vi "Hardware Config - format and values.vi"(11 "Hardware Configuration":T4={"Dev. PC"=FALSE, "Swap XY on stage"=FALSE, "No of AOD"=0, "Computer MAC address"="", "Externalise Triggers"=FALSE, "Trigger HW config"={"Available Device List"=0, "Device Address"=""}, "DAQmx Chan"={"Pockels AO"="", "Hard shutter AO"="", "PMT AOs"="", "Galvo AOs"="", "Power meter AI"=""}, "XY stage available"=FALSE, "XY Stage"={"COM port"="", "Baudrate"=0, "Type"=""}, "Z stage available"=FALSE, "Z Stage config cluster"={"COM port"="COM7", "Baudrate"=0, "Type"=""}, "Encoder available"=FALSE, "Encoder"={"IP address"="224.0.1.103", "Port"=7000, "Wheel radius (cm)"=16.0, "Encoder Trigger"=""}, "VidRec available"=FALSE, "Cam VidRec"={"DO flag-Video record"="", "DO flag-Trial start"=""}, "Laser Power Control HW config"={"Laser Power Control"="", "Laser Power Modulation Control"=enum."NI"}, "Laser 1 available"=FALSE, "Laser 1 config cluster"={"COM port"="COM7", "Baud Rate"=0, "Type"=""}, "Prechirper 1 available"=FALSE, "Prechirper 1 config cluster"={"Type"="", "Baud Rate"=0, "COM port"="COM7"}, "Control system.FPGA available?"=FALSE, "Control Sys. HW config"={"Control system.FPGA Type"=enum."Virtex 5", "Control system.Network adapter name"="", "Control system.MAC address"="", "Control system.Ethernet Port"=0, "Control system.Ethernet Port Opened"=FALSE}, "DAQ FPGA HW Config"={"FGPA Ref"=refnum, "Target"="RIO0", "input card type"=enum."AC Card"}} {"Encoder"."Wheel radius (cm)" format="%#_13g"}) -> (0 "String":string[](array[string]), 1 "String":T1, 2 "Numeric":dbl[](array[numeric]), 3 "Numeric":T3=[{"key"="Encoder.Port", "Save?"=TRUE, "Default"=7000.0}, {"key"="Encoder.Wheel radius (cm)", "Save?"=TRUE, "Default"=16.0}, {"key"="DAQ FPGA.Input type AC/DC", "Save?"=TRUE, "Default"=1.0}, {"key"="Num AOD", "Save?"=TRUE, "Default"=4.0}, {"key"="Trigger.AvailableDeviceList", "Save?"=TRUE, "Default"=1.0}, {"key"="XY Stage.Baudrate", "Save?"=TRUE, "Default"=9600.0}, {"key"="Z Stage.Baudrate", "Save?"=TRUE, "Default"=9600.0}, {"key"="Laser.Baudrate", "Save?"=TRUE, "Default"=19200.0}, {"key"="Prechirper.Baudrate", "Save?"=TRUE, "Default"=115200.0}], 4 "Boolean":bool[](array[boolean]), 6 "Boolean":T2=[{"key"="DevPC - No hardware", "Save?"=TRUE, "Default"=FALSE}, {"key"="MC Supported", "Save?"=TRUE, "Default"=FALSE}, {"key"="Axial MC", "Save?"=TRUE, "Default"=FALSE}, {"key"="Are X Y Swapped", "Save?"=TRUE, "Default"=FALSE}, {"key"="Encoder.Available?", "Save?"=TRUE, "Default"=FALSE}, {"key"="Externalise Triggers", "Save?"=TRUE, "Default"=TRUE}, {"key"="Cam VidRec.Available", "Save?"=TRUE, "Default"=TRUE}, {"key"="Control system.Ctrl FPGA available", "Save?"=TRUE, "Default"=TRUE}, {"key"="XY Stage.Available?", "Save?"=TRUE, "Default"=TRUE}, {"key"="Z Stage.Available?", "Save?"=TRUE, "Default"=FALSE}, {"key"="Laser.Available?", "Save?"=TRUE, "Default"=TRUE}, {"key"="Prechirper.Available", "Save?"=TRUE, "Default"=TRUE}])   [LabVIEW 2017]
uses:
  Typedefs/Hardware Configuration settings.ctl
  Typedefs/Triggers HW config.ctl
  Typedefs/DAQmx physical channels cluster.ctl
  Typedefs/XY Stage config cluster.ctl
  Typedefs/Z Stage config cluster.ctl
  Typedefs/Encoder config cluster.ctl
  Typedefs/Cam VidRec HW config setup cluster.ctl
  Typedefs/Laser Power Control HW config.ctl
  Typedefs/Laser 1 config cluster.ctl
  Typedefs/PreChirper 1 config cluster.ctl
  Typedefs/Control Sys HW config cluster.ctl
  Typedefs/DAQ FPGA HW config cluster.ctl
  RIG-SPECIFIC FILES/FPGA Refs/FPGA Ref.ctl
  <vilib>/userdefined/High Color/nirio_resource_hc.ctl
  Typedefs/FPGA input type AC-DC.ctl
  Typedefs/Ini file interface (DBL).ctl
  Typedefs/Ini file interface (Boolean).ctl
  Typedefs/Ini file interface (String).ctl
panel:
  out "Boolean Default cluster":i32
  out "Boolean values":i32
  out "Numeric Values":i32
  out "Numeric Default Cluster":i32
  out "String values":i32
  out "String Default Cluster":i32
  # "Numeric Array Sizes"
  # "String Array Sizes"
  # "Boolean Array Sizes"
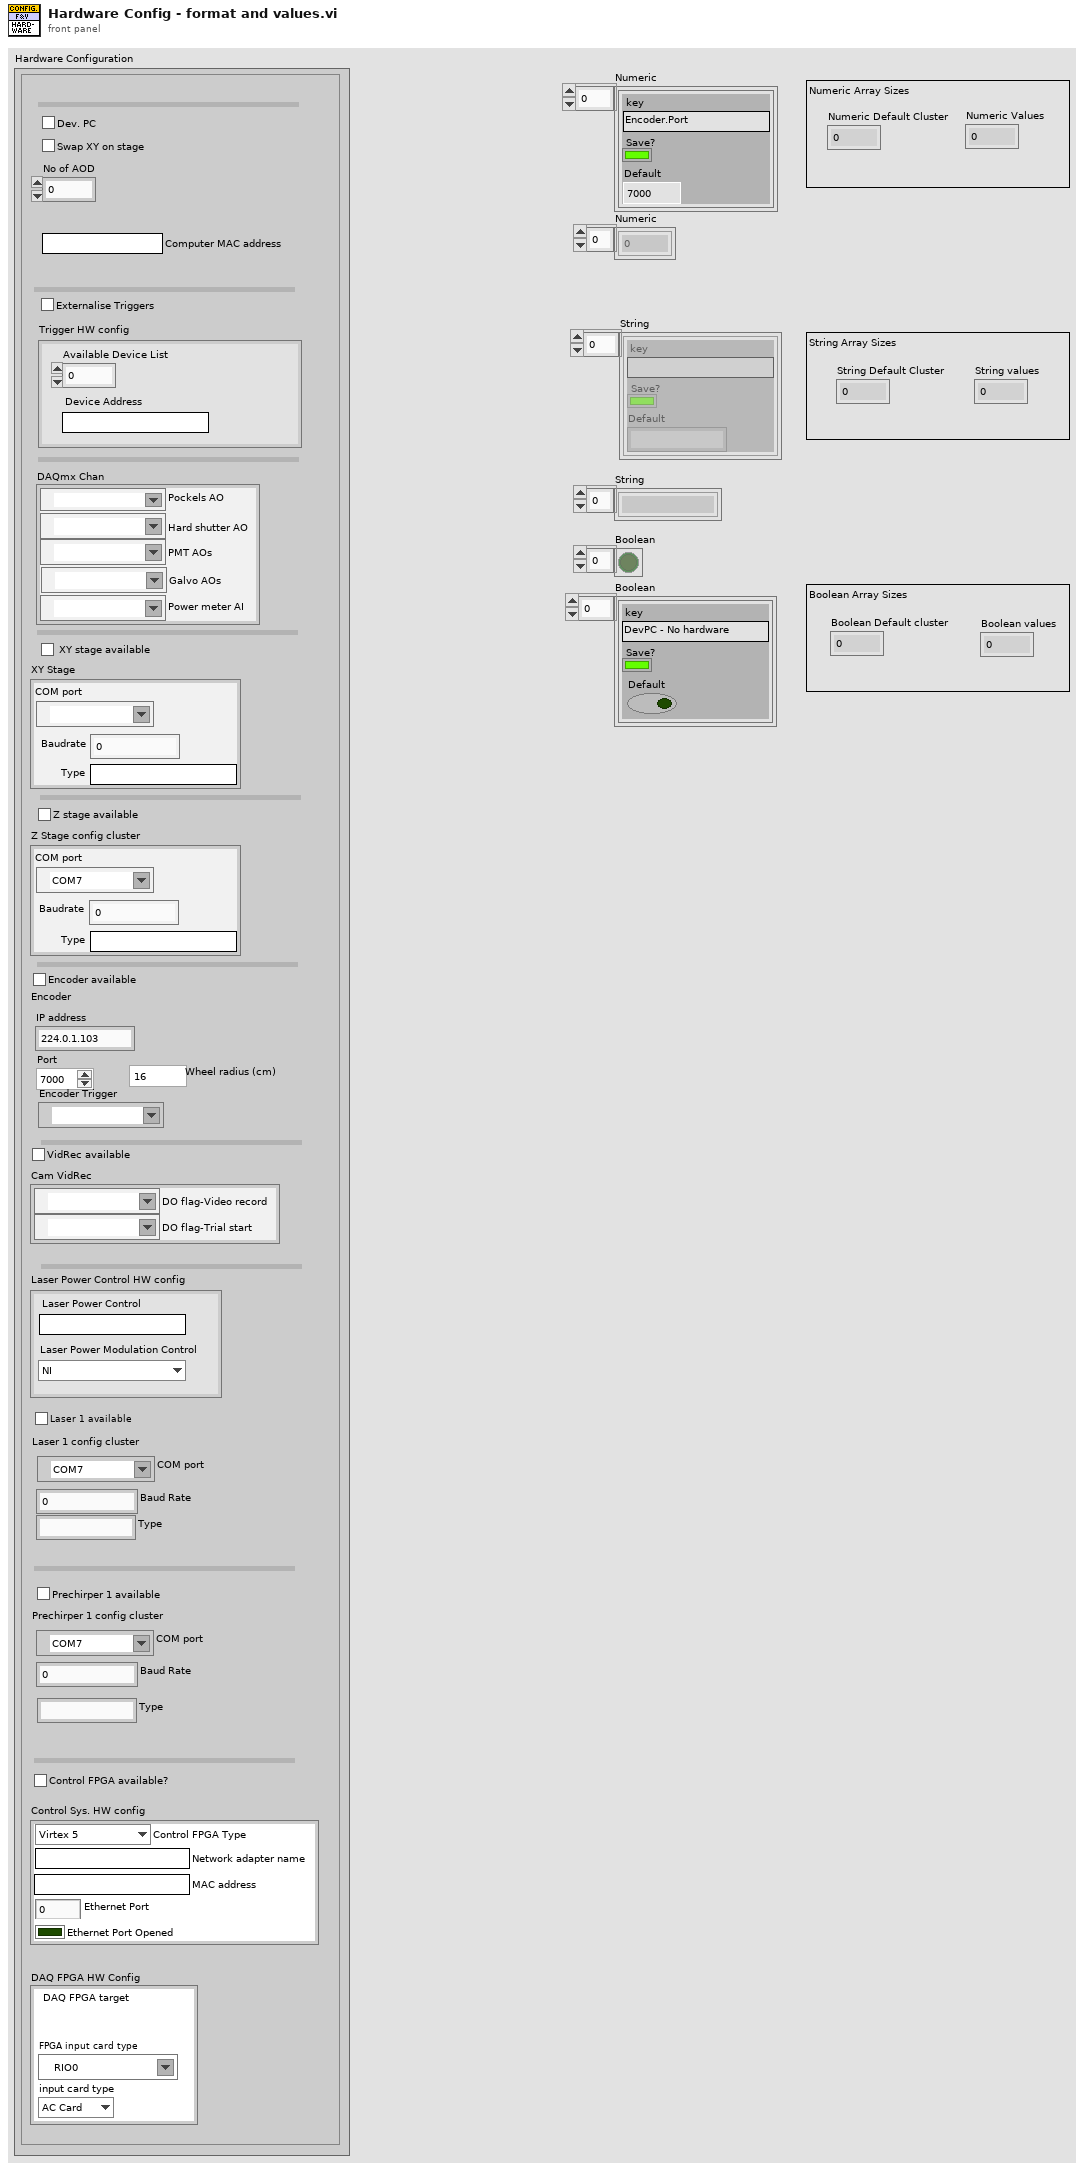
[diagram p1: front panel]
types:
  T1 = typedef "Ini file interface (String).ctl" = cluster{"key":string, "Save?":bool, "Default":string}[]
  T2 = typedef "Ini file interface (Boolean).ctl" = cluster{"key":string, "Save?":bool, "Default":bool}[]
  T3 = typedef "Ini file interface (DBL).ctl" = cluster{"key":string, "Save?":bool, "Default":dbl}[]
  T4 = typedef "Hardware Configuration settings.ctl" = cluster{"Dev. PC":bool, "Swap XY on stage":bool, "No of AOD":u8, "Computer MAC address":string, "Externalise Triggers":bool, "Trigger HW config":T5, "DAQmx Chan":T6, "XY stage available":bool, "XY Stage":T7, "Z stage available":bool, "Z Stage config cluster":T8, "Encoder available":bool, "Encoder":T9, "VidRec available":bool, "Cam VidRec":T10, "Laser Power Control HW config":T11, "Laser 1 available":bool, "Laser 1 config cluster":T12, "Prechirper 1 available":bool, "Prechirper 1 config cluster":T13, "Control system.FPGA available?":bool, "Control Sys. HW config":T14, "DAQ FPGA HW Config":T15}
  T5 = typedef "Triggers HW config.ctl" = cluster{"Available Device List":i32, "Device Address":string}
  T6 = typedef "DAQmx physical channels cluster.ctl" = cluster{"Pockels AO":tag, "Hard shutter AO":tag, "PMT AOs":tag, "Galvo AOs":tag, "Power meter AI":tag}
  T7 = typedef "XY Stage config cluster.ctl" = cluster{"COM port":refnum<visa-resource-name>, "Baudrate":i32, "Type":string}
  T8 = typedef "Z Stage config cluster.ctl" = cluster{"COM port":refnum<visa-resource-name>, "Baudrate":i32, "Type":string}
  T9 = typedef "Encoder config cluster.ctl" = cluster{"IP address":string, "Port":u16, "Wheel radius (cm)":dbl, "Encoder Trigger":tag}
  T10 = typedef "Cam VidRec HW config setup cluster.ctl" = cluster{"DO flag-Video record":tag, "DO flag-Trial start":tag}
  T11 = typedef "Laser Power Control HW config.ctl" = cluster{"Laser Power Control":string, "Laser Power Modulation Control":enum16{"NI", "FPGA"}}
  T12 = typedef "Laser 1 config cluster.ctl" = cluster{"COM port":refnum<visa-resource-name>, "Baud Rate":i32, "Type":string}
  T13 = typedef "PreChirper 1 config cluster.ctl" = cluster{"Type":string, "Baud Rate":i32, "COM port":refnum<visa-resource-name>}
  T14 = typedef "Control Sys HW config cluster.ctl" = cluster{"Control system.FPGA Type":enum16{"Virtex 5", "Virtex 7"}, "Control system.Network adapter name":string, "Control system.MAC address":string, "Control system.Ethernet Port":u32, "Control system.Ethernet Port Opened":bool}
  T15 = typedef "DAQ FPGA HW config cluster.ctl" = cluster{"FGPA Ref":T16, "Target":T17, "input card type":T18}
  T16 = typedef "FPGA Ref.ctl" = refnum<k20>
  T17 = typedef "nirio_resource_hc.ctl" = tag
  T18 = typedef "FPGA input type AC-DC.ctl" = enum16{"AC Card", "DC Card"}
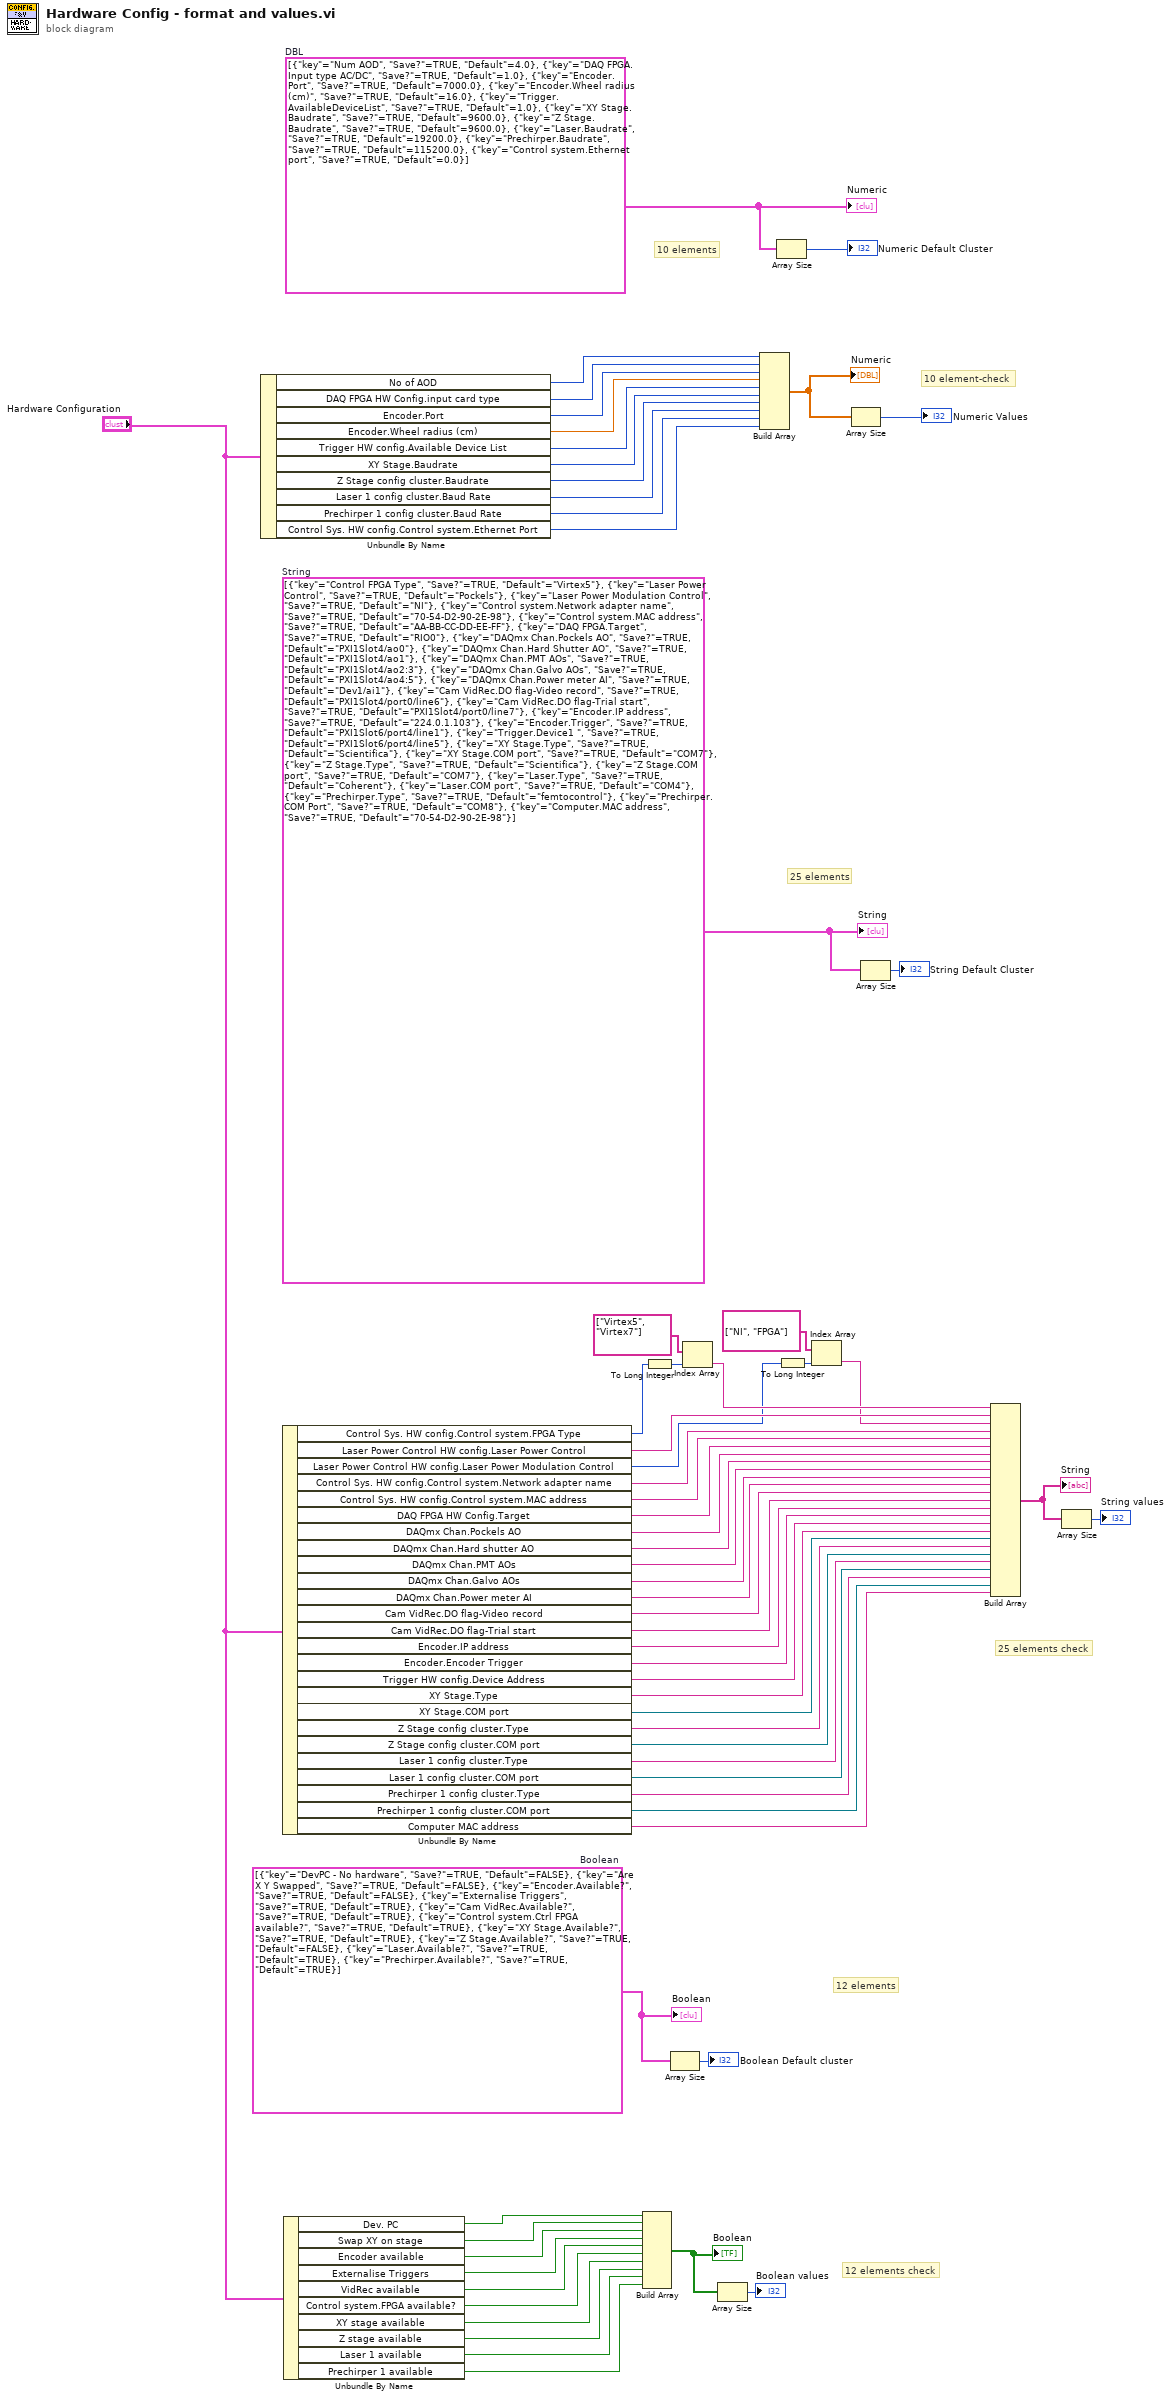
[diagram p0: block diagram]
diagram:
  w12 = T2 [{"key"="DevPC - No hardware", "Save?"=TRUE, "Default"=FALSE}, {"key"="Are X Y Swapped", "Save?"=TRUE, "Default"=FALSE}, {"key"="Encoder.Available?", "Save?"=TRUE, "Default"=FALSE}, {"key"="Externalise Triggers", "Save?"=TRUE, "Default"=TRUE}, {"key"="Cam VidRec.Available?", "Save?"=TRUE, "Default"=TRUE}, {"key"="Control system.Ctrl FPGA available?", "Save?"=TRUE, "Default"=TRUE}, {"key"="XY Stage.Available?", "Save?"=TRUE, "Default"=TRUE}, {"key"="Z Stage.Available?", "Save?"=TRUE, "Default"=FALSE}, {"key"="Laser.Available?", "Save?"=TRUE, "Default"=TRUE}, {"key"="Prechirper.Available?", "Save?"=TRUE, "Default"=TRUE}]  # Boolean
  w22 = T1 [{"key"="Control FPGA Type", "Save?"=TRUE, "Default"="Virtex5"}, {"key"="Laser Power Control", "Save?"=TRUE, "Default"="Pockels"}, {"key"="Laser Power Modulation Control", "Save?"=TRUE, "Default"="NI"}, {"key"="Control system.Network adapter name", "Save?"=TRUE, "Default"="70-54-D2-90-2E-98"}, {"key"="Control system.MAC address", "Save?"=TRUE, "Default"="AA-BB-CC-DD-EE-FF"}, {"key"="DAQ FPGA.Target", "Save?"=TRUE, "Default"="RIO0"}, {"key"="DAQmx Chan.Pockels AO", "Save?"=TRUE, "Default"="PXI1Slot4/ao0"}, {"key"="DAQmx Chan.Hard Shutter AO", "Save?"=TRUE, "Default"="PXI1Slot4/ao1"}, {"key"="DAQmx Chan.PMT AOs", "Save?"=TRUE, "Default"="PXI1Slot4/ao2:3"}, {"key"="DAQmx Chan.Galvo AOs", "Save?"=TRUE, "Default"="PXI1Slot4/ao4:5"}, {"key"="DAQmx Chan.Power meter AI", "Save?"=TRUE, "Default"="Dev1/ai1"}, {"key"="Cam VidRec.DO flag-Video record", "Save?"=TRUE, "Default"="PXI1Slot4/port0/line6"}, {"key"="Cam VidRec.DO flag-Trial start", "Save?"=TRUE, "Default"="PXI1Slot4/port0/line7"}, {"key"="Encoder.IP address", "Save?"=TRUE, "Default"="224.0.1.103"}, {"key"="Encoder.Trigger", "Save?"=TRUE, "Default"="PXI1Slot6/port4/line1"}, {"key"="Trigger.Device1 ", "Save?"=TRUE, "Default"="PXI1Slot6/port4/line5"}, {"key"="XY Stage.Type", "Save?"=TRUE, "Default"="Scientifica"}, {"key"="XY Stage.COM port", "Save?"=TRUE, "Default"="COM7"}, {"key"="Z Stage.Type", "Save?"=TRUE, "Default"="Scientifica"}, {"key"="Z Stage.COM port", "Save?"=TRUE, "Default"="COM7"}, {"key"="Laser.Type", "Save?"=TRUE, "Default"="Coherent"}, {"key"="Laser.COM port", "Save?"=TRUE, "Default"="COM4"}, {"key"="Prechirper.Type", "Save?"=TRUE, "Default"="femtocontrol"}, {"key"="Prechirper.COM Port", "Save?"=TRUE, "Default"="COM8"}, {"key"="Computer.MAC address", "Save?"=TRUE, "Default"="70-54-D2-90-2E-98"}]  # String
  w17 = T3 [{"key"="Num AOD", "Save?"=TRUE, "Default"=4.0}, {"key"="DAQ FPGA.Input type AC/DC", "Save?"=TRUE, "Default"=1.0}, {"key"="Encoder.Port", "Save?"=TRUE, "Default"=7000.0}, {"key"="Encoder.Wheel radius (cm)", "Save?"=TRUE, "Default"=16.0}, {"key"="Trigger.AvailableDeviceList", "Save?"=TRUE, "Default"=1.0}, {"key"="XY Stage.Baudrate", "Save?"=TRUE, "Default"=9600.0}, {"key"="Z Stage.Baudrate", "Save?"=TRUE, "Default"=9600.0}, {"key"="Laser.Baudrate", "Save?"=TRUE, "Default"=19200.0}, {"key"="Prechirper.Baudrate", "Save?"=TRUE, "Default"=115200.0}, {"key"="Control system.Ethernet port", "Save?"=TRUE, "Default"=0.0}]  # DBL
  # "12 elements check"
  # "12 elements"
  # "25 elements check"
  # "25 elements"
  # "10 element-check"
  # "10 elements"
  n1 = Unbundle By Name("Hardware Configuration") -> ("No of AOD"=w32:u8, "DAQ FPGA HW Config.input card type"=w31:T18, "Encoder.Port"=w30:u16, "Encoder.Wheel radius (cm)"=w29:dbl, "Trigger HW config.Available Device List"=w28:i32, "XY Stage.Baudrate"=w27:i32, "Z Stage config cluster.Baudrate"=w26:i32, "Laser 1 config cluster.Baud Rate"=w25:i32, "Prechirper 1 config cluster.Baud Rate"=w24:i32, "Control Sys. HW config.Control system.Ethernet Port"=w1:u32)
  n2 = Unbundle By Name("Hardware Configuration") -> ("Control Sys. HW config.Control system.FPGA Type"=w9:enum16{"Virtex 5", "Virtex 7"}, "Laser Power Control HW config.Laser Power Control"=w64:string, "Laser Power Control HW config.Laser Power Modulation Control"=w5:enum16{"NI", "FPGA"}, "Control Sys. HW config.Control system.Network adapter name"=w63:string, "Control Sys. HW config.Control system.MAC address"=w62:string, "DAQ FPGA HW Config.Target"=w33:T17, "DAQmx Chan.Pockels AO"=w61:tag, "DAQmx Chan.Hard shutter AO"=w60:tag, "DAQmx Chan.PMT AOs"=w59:tag, "DAQmx Chan.Galvo AOs"=w23:tag, "DAQmx Chan.Power meter AI"=w58:tag, "Cam VidRec.DO flag-Video record"=w57:tag, "Cam VidRec.DO flag-Trial start"=w56:tag, "Encoder.IP address"=w55:string, "Encoder.Encoder Trigger"=w54:tag, "Trigger HW config.Device Address"=w53:string, "XY Stage.Type"=w52:string, "XY Stage.COM port"=w51:refnum<visa-resource-name>, "Z Stage config cluster.Type"=w50:string, "Z Stage config cluster.COM port"=w49:refnum<visa-resource-name>, "Laser 1 config cluster.Type"=w48:string, "Laser 1 config cluster.COM port"=w47:refnum<visa-resource-name>, "Prechirper 1 config cluster.Type"=w46:string, "Prechirper 1 config cluster.COM port"=w45:refnum<visa-resource-name>, "Computer MAC address"=w2:string)
  n3 = Unbundle By Name("Hardware Configuration") -> ("Dev. PC"=w43:bool, "Swap XY on stage"=w42:bool, "Encoder available"=w41:bool, "Externalise Triggers"=w40:bool, "VidRec available"=w39:bool, "Control system.FPGA available?"=w38:bool, "XY stage available"=w37:bool, "Z stage available"=w36:bool, "Laser 1 available"=w35:bool, "Prechirper 1 available"=w34:bool)
  n4 = Build Array(w43, w42, w41, w40, w39, w38, w37, w36, w35, w34) -> (w11:bool[])
  "Boolean" <- w11
  n5 = To Long Integer(number=w9) -> (32bit integer=w8:i32)
  n6 = Array Size(array=w12) -> (size(s)=→"Boolean Default cluster":i32)
  n7 = Index Array(array=string[] ["Virtex5", "Virtex7"], index=w8) -> (element=w7:string)
  n8 = Array Size(array=w11) -> (size(s)=→"Boolean values":i32)
  n9 = Build Array(w32, w31, w30, w29, w28, w27, w26, w25, w24, w1) -> (w15:dbl[])
  "Numeric" <- w15
  n10 = Array Size(array=w17) -> (size(s)=→"Numeric Default Cluster":i32)
  n11 = To Long Integer(number=w5) -> (32bit integer=w4:i32)
  n12 = Index Array(array=string[] ["NI", "FPGA"], index=w4) -> (element=w3:string)
  n13 = Array Size(array=w15) -> (size(s)=→"Numeric Values":i32)
  n14 = Array Size(array=w22) -> (size(s)=→"String Default Cluster":i32)
  n15 = Build Array(w7, w64, w3, w63, w62, w33, w61, w60, w59, w23, w58, w57, w56, w55, w54, w53, w52, w51, w50, w49, w48, w47, w46, w45, w2) -> (w19:string[])
  "String" <- w19
  n16 = Array Size(array=w19) -> (size(s)=→"String values":i32)
  "Numeric" <- w17
  "Boolean" <- w12
  "String" <- w22
